vi "15-SetInitialPosition.vi"(9 "Initial Position in":cluster{"Row":i32, "Col":i32}, 10 "map in":T1(c390), 11 "Visited Array in":bool[][](array[boolean])) -> (1 "Initial Position out":cluster{"Row":i32, "Col":i32}, 2 "map out":T1(c390), 3 "Visited Array out":bool[][](array[boolean]))   [LabVIEW 2019, in "15.lvlib"]
uses:
  15.lvlib
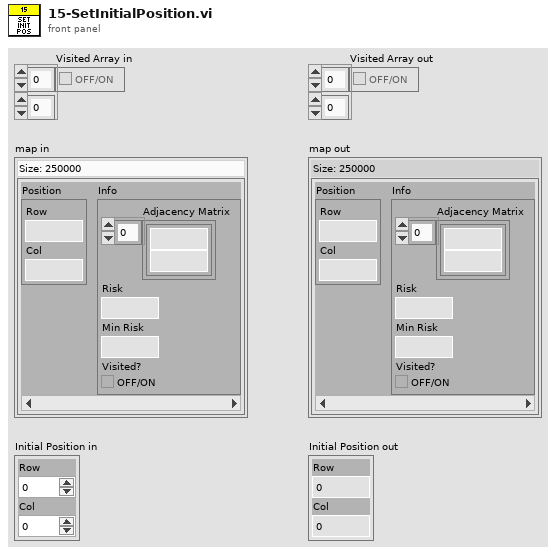
[diagram p1: front panel]
types:
  T1 = map{cluster{"Row":i32, "Col":i32}, cluster{"Adjacency Matrix":cluster{i32, i32}[], "Risk":u8, "Min Risk":i32, "Visited?":bool}}
  T2 = cluster{"Adjacency Matrix":cluster{i32, i32}[], "Cost":u8, "Min Cost":i32, "Visited?":bool}
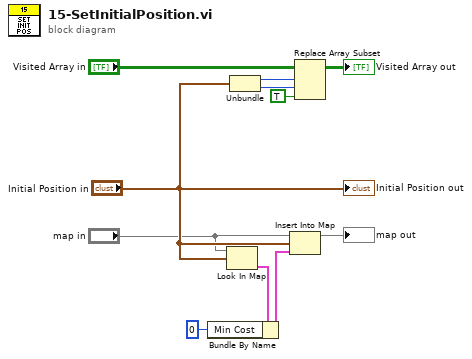
[diagram p0: block diagram]
diagram:
  n1 = Look In Map(map="map in", key="Initial Position in") -> (value=w9:T2)  [unwired: 1 in, 1 out]
  n2 = Bundle By Name(cluster=w9, "Min Cost"=u32 0) -> (w10:T2)
  n3 = Unbundle("Initial Position in") -> ("Row"=w2:i32, "Col"=w4:i32)
  n4 = Insert Into Map(map in="map in", key="Initial Position in", value=w10) -> (map out=→"map out":T1)  [unwired: 2 out]
  n5 = Replace Array Subset(array="Visited Array in", new element=TRUE ("new element/subarray"), index (row)=w2, index (col)=w4) -> (→"Visited Array out":bool[][])
  "Initial Position out" <- "Initial Position in"
